vi "AcquireImage.vi"(6 "Image Conversion":string, 7 "measure call context in":refnum<class "Measure Call Context.lvclass">, 8 "error in (no error)":errorcluster, 9 "Buffer Number Out in":u32, 10 "Accessor:Is Canceled":bool, 11 "Refnum in":T2) -> (0 "error out":errorcluster, 1 "Valid Result":bool, 2 "Measurement Results":T1, 3 "Buffer Number Out out":u32)   [LabVIEW 2021, in "ImageRendering.lvlib"]
uses:
  ImageRendering.lvlib
  <vilib>/userdefined/High Color/IMAQdx.ctl
  <vilib>/MeasurementLink/MeasurementLink Measurement Server/Measure Call Context/Measure Call Context.lvclass
  Measurement Results.ctl
  <resource>/objmgr/imaqdx.rc
  <vilib>/vision/driver/NI_Vision_Acquisition_Software.lvlib
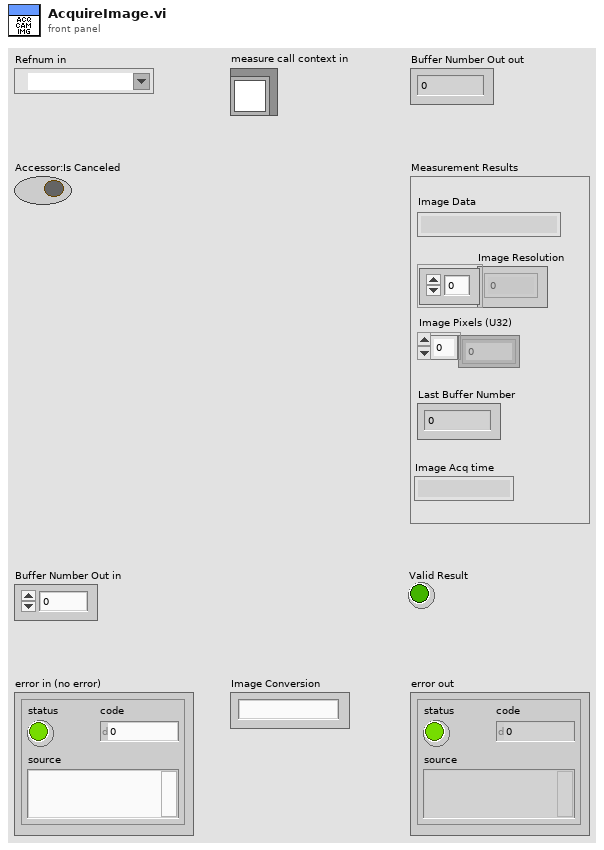
[diagram p1: front panel]
types:
  T1 = typedef "ImageRendering.lvlib/Measurement Results.ctl" = cluster{"Image Data":string, "Image Resolution":i32[], "Image Pixels (U32)":u32[], "Last Buffer Number":u32, "Image Acq time":string}
  T2 = typedef "IMAQdx.ctl" = refnum<k21>
  T3 = typedef "IMAQ Image.ctl" = refnum<image>
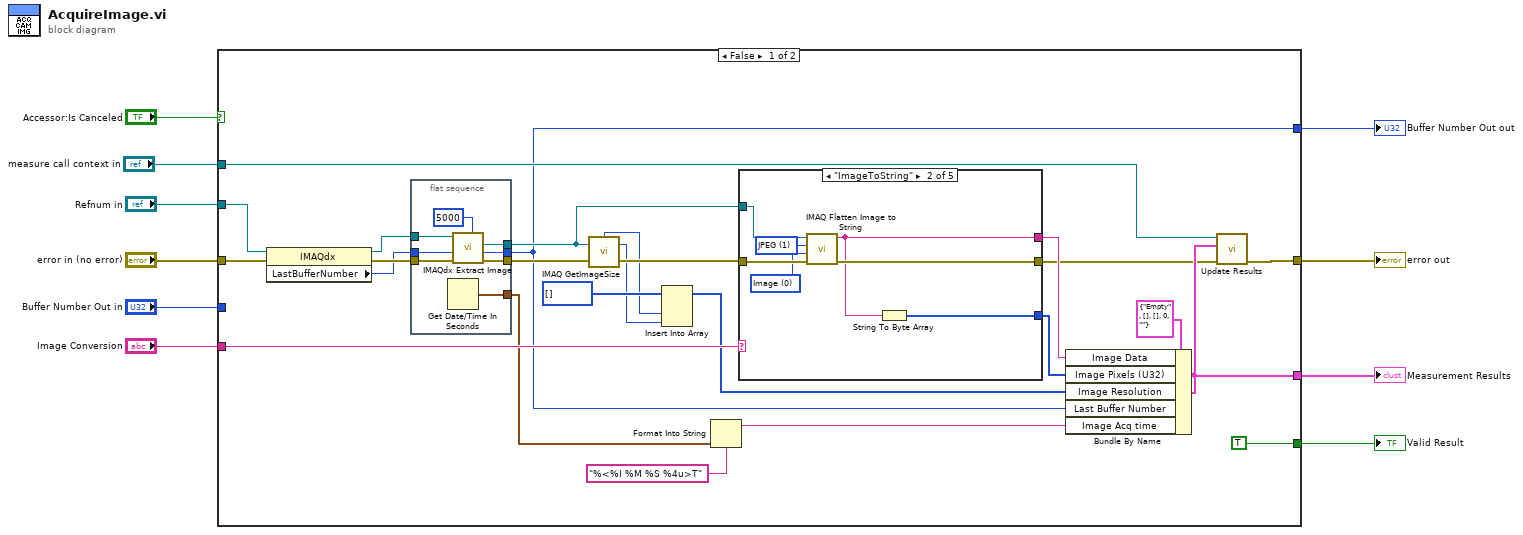
[diagram p0: block diagram]
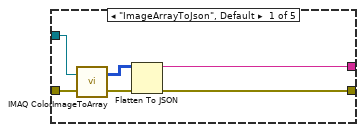
[diagram p2: hidden frame]
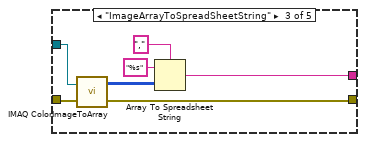
[diagram p3: hidden frame]
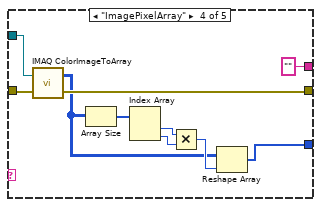
[diagram p4: hidden frame]
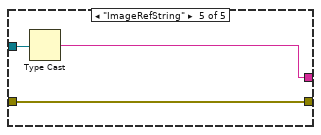
[diagram p5: hidden frame]
diagram:
  n1 = case shown="False" "Accessor:Is Canceled" {
    tunnel: "Refnum in" -> [w35 _]
    tunnel: [w32 w77] -> w6
    tunnel: [w14 w78] -> w7
    tunnel: "Buffer Number Out in" -> [_ w78]
    tunnel: "error in (no error)" -> [w30 w77]
    tunnel: "Image Conversion" -> [w29 _]
    tunnel: [w28 _] -> w2
    tunnel: "measure call context in" -> [w27 _]
    tunnel: [TRUE _] -> w1
    frame False {
      n2 = property class="IMAQdx"(reference=w35, error in=w30) -> (reference out=w34:T2, error out=w33:errorcluster, "LastBufferNumber"=w31:u32)
      n3 = flat-sequence {
        tunnel: w34 -> [w43]
        tunnel: w33 -> [w42]
        tunnel: w31 -> [w41]
        tunnel: [w39] -> w22
        tunnel: [w38] -> w20
        tunnel: [w37] -> w14
        tunnel: [w36] -> w13
        frame #0 {
          n4 = Get Date/Time In Seconds() -> (seconds since 1Jan1904=w36:timestamp)
          n5 = call <vilib>:"IMAQdx Extract Image.vi"("Timeout (ms)"=5000, "error in"=w42, "Buffer Number In"=w41, "Session In"=w43) -> ("error out"=w39:errorcluster, "Buffer Number Out"=w37:u32, "Image Out"=w38:T3)  [unwired: 4 in, 1 out]
        }
      }
      n6 = call "IMAQ GetImageSize"("Image"=w20, "error in (no error)"=w22) -> ("Y Resolution"=w16:i32, "X Resolution"=w17:i32, "error out"=w21:errorcluster)  [unwired: 2 in]
      n7 = Insert Into Array(array=i32[] [] ("size(s)"), new element #1=w17, new element #2=w16) -> (w15:i32[])  [unwired: 1 in]
      n8 = Format Into String(format string="%<%I %M %S %4u>T", w13) -> (resulting string=w11:string)  [unwired: 2 in, 1 out]
      n9 = case shown="\"ImageToString\"" w29 {
        tunnel: w21 -> [w49 w56 w63 w73 w76]
        tunnel: [w47 w55 w62 w72 w76] -> w19
        tunnel: [w46 w52 w59 "" ("spreadsheet string") w74] -> w24
        tunnel: w20 -> [w44 w53 w57 w70 w75]
        tunnel: [_ w51 _ w64 _] -> w23
        frame "ImageArrayToJson", Default {
          n10 = call "IMAQ ColorImageToArray"("Image"=w44, "error in (no error)"=w49) -> ("Image Pixels (U32)"=w45:u32[][], "error out"=w48:errorcluster)  [unwired: 2 in, 1 out]
          n11 = Flatten To JSON(anything=w45, error in (no error)=w48) -> (JSON string=w46:string, 11:w47:errorcluster)  [unwired: 1 in]
        }
        frame "ImageToString" {
          w50 = 1 items=["None", "JPEG", "PACKED BINARY"] ("Compression (None)")
          w54 = 0 items=["Image", "Image and Vision Info", "Reference to Image"] ("Type of Flatten (Image and Vision Info)")
          n12 = call "IMAQ Flatten Image to String"("error in (no error)"=w56, "Type of Flatten (Image and Vision Info)"=w54, "Compression (None)"=w50, "Image"=w53) -> ("error out"=w55:errorcluster, "Data String"=w52:string)  [unwired: 6 in]
          n13 = String To Byte Array(string=w52) -> (unsigned byte array=w51:u8[])
        }
        frame "ImageArrayToSpreadSheetString" {
          n14 = call "IMAQ ColorImageToArray"("Image"=w57, "error in (no error)"=w63) -> ("Image Pixels (U32)"=w61:u32[][], "error out"=w62:errorcluster)  [unwired: 2 in, 1 out]
          n15 = Array To Spreadsheet String(delimiter (Tab)=",", array=w61, 3:"%s" ("format string")) -> (spreadsheet string=w59:string)
        }
        frame "ImagePixelArray" {
          n16 = call "IMAQ ColorImageToArray"("Image"=w70, "error in (no error)"=w73) -> ("Image Pixels (U32)"=w66:u32[][], "error out"=w72:errorcluster)  [unwired: 2 in, 1 out]
          n17 = Array Size(array=w66) -> (size(s)=w65:i32[])
          n18 = Index Array(array=w65) -> (element #1=w69:i32, element #2=w68:i32)  [unwired: 2 in]
          n19 = Multiply(x=w69, y=w68) -> (x*y=w67:i32)
          n20 = Reshape Array(w66, w67) -> (w64:u32[])
        }
        frame "ImageRefString" {
          n21 = Type Cast(x=w75) -> (*(type *) &x=w74:string)  [unwired: 1 in]
        }
      }
      n22 = Bundle By Name(cluster=T1 {"Image Data"="Empty", "Image Resolution"=[], "Image Pixels (U32)"=[], "Last Buffer Number"=0, "Image Acq time"=""} ("Measurement Results"), "Image Data"=w24, "Image Pixels (U32)"=w23, "Image Resolution"=w15, "Last Buffer Number"=w14, "Image Acq time"=w11) -> (w28:T1)
      n23 = call <vilib>:"Update Results.vi"("error in"=w19, "measurement results"=w28, "measure call context in"=w27) -> ("error out"=w32:errorcluster)  [unwired: 7 in, 1 out]
    }
    frame True {
    }
  }
  "Buffer Number Out out" <- w7
  "error out" <- w6
  "Measurement Results" <- w2
  "Valid Result" <- w1
